vi "PH_PowerUnit_BaseClass.PC_EnablingState.vi"(0 "i ref in":refnum<vi>, 2 "Tagvalue":i32, 5 "error in (no error)":errorcluster) -> (14 "i ref out":refnum<vi>, 19 "error out":errorcluster)   [LabVIEW 2014, in "PH_PowerUnit_BaseClass.lvlib"]
doc: "This VI writes the Information from the PA Enabling Tag to own attributes and sets the GUI object."
uses:
  PH_PowerUnit_BaseClass.lvlib
  PH_SystemInformation/PH_SystemInformationEnabling State.ctl
  PH_SystemInformation/PH_SystemInformation.lvlib
  PH_Common/PH_Common.lvlib
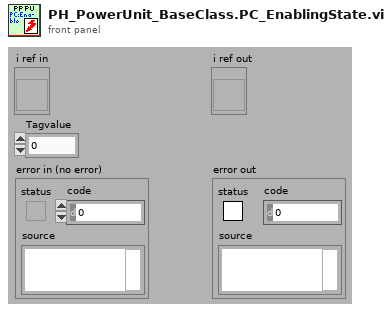
[diagram p1: front panel]
types:
  T1 = typedef "PH_PowerUnit_BaseClass.lvlib/PH_PowerUnit_BaseClass.i attribute.ctl" = cluster{"Constructor finished":bool, "PU":cluster{"In use":bool, "Service ID in use":i32, "GUI Ref":refnum<vi>}, "Enabling":cluster{"State":T2, "GUI Ref":refnum<vi>}, "Timing":cluster{"Last Shot":dbl, "Time between Shots [Sec]":dbl, "Waiting Time over?":bool, "Service ID Waiting Time":i32, "GUI Ref":refnum<vi>, "Instance":cluster{"Status":T3, "linked?":bool, "GUI Ref":refnum<vi>}}, "Sequencer":cluster{"SM State":string, "GUI Ref":refnum<vi>, "linked":bool}, "Subscribed Trendmssgs":cluster{"Tagname":string, "Status":T3, "linked?":bool, "Shot Condition":T3, "GUI Ref":refnum<vi>}[], "PP PU":T4, "Default Voltage (V)":dbl, "GUI Refs":T5, "PSDB data":cluster{"Shot Voltage [V]":dbl, "State TO SM":T6, "Write 2 early":bool}, "State TO SM":T6}
  T2 = typedef "PH_SystemInformation.lvlib/PH_SystemInformationEnabling State.ctl" = i32
  T3 = typedef "PH_StatusHandler.lvlib/PH_StatusHandler.Status.ctl" = i16
  T4 = typedef "PH_PP_Common.lvlib/PH_PP_Common.PUs.ctl" = enum16{"no Info", "PA-19mm-1", "PA-19mm-2", "PA-45mm-PILC", "PA-45mm-MAIN", "MA-PU-1", "MA-PU-2", "MA-PU-3", "MA-PU-4", "MA-PU-5", "MA-PU-6", "MA-FR", "MA-PILC", "PA-45mm-DP"}
  T5 = typedef "PH_PowerUnit_BaseClass.lvlib/PH_PowerUnit_BaseClass.GUI Refs.ctl" = cluster{"Delete Inst":refnum<vi>, "State TO SM":refnum<vi>, "State SM":refnum<vi>, "Fire":refnum<vi>}
  T6 = typedef "PH_PowerUnit_BaseClass.lvlib/PH_PowerUnit_BaseClass.SM States.ctl" = enum16{".", "Stand by", "Switch PU on", "Configure", "Set Default Voltage", "Set STANDBY", "Set READY", "Wait for Shot Cmd", "Open Dump Rods", "Open Ross Relais", "Close Ross Relais", "Switch PSU on", "Switch PSU off", "Charge", "Switch GD Channel on", "Close Dump Rods", "Rods-TO", "RR-TO", "PSU-TO", "Trigger-TO"}
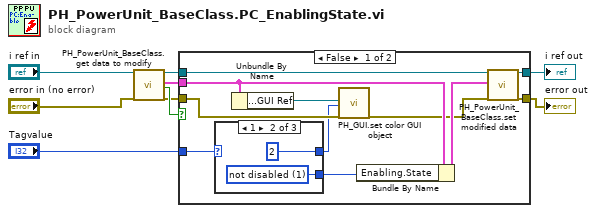
[diagram p0: block diagram]
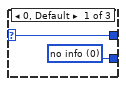
[diagram p2: hidden frame]
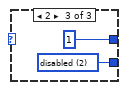
[diagram p3: hidden frame]
diagram:
  n1 = call "PH_PowerUnit_BaseClass.get data to modify.vi"("i ref in"="i ref in", "error in (no error)"="error in (no error)") -> ("i ref out"=w3:refnum<vi>, "i attribute"=w2:T1, "timed out"=w9:bool, "error out"=w5:errorcluster)  [unwired: 14 in]
  n2 = case shown="False" w9 {
    tunnel: w3 -> [w20 w28]
    tunnel: [w15 w28] -> w4
    tunnel: w5 -> [w12 w27]
    tunnel: [w14 w27] -> w6
    tunnel: w2 -> [w18 _]
    tunnel: "Tagvalue" -> [w17 _]
    frame False {
      n3 = case shown="1" w17 {
        selector: w17 -> [w22 _ _]
        tunnel: [w22 2 1 ("Numeric")] -> w10
        tunnel: [w21 w23 w25] -> w16
        frame 0, Default {
          w21 = T2 0 items=["no info", "not disabled", "disabled"] ("MainAmp Enabling State")
        }
        frame 1 {
          w23 = T2 1 items=["no info", "not disabled", "disabled"] ("MainAmp Enabling State")
        }
        frame 2 {
          w25 = T2 2 items=["no info", "not disabled", "disabled"] ("MainAmp Enabling State")
        }
      }
      n4 = Unbundle By Name(w18) -> ("Enabling.GUI Ref"=w13:refnum<vi>)
      n5 = call "PH_GUI.set color GUI object.vi"("GUI object Ref"=w13, "State"=w10, "error in (no error)"=w12) -> ("error out"=w11:errorcluster)  [unwired: 16 in]
      n6 = Bundle By Name(cluster=w18, "Enabling.State"=w16) -> (w19:T1)
      n7 = call "PH_PowerUnit_BaseClass.set modified data.vi"("i ref in"=w20, "i attribute"=w19, "error in (no error)"=w11) -> ("i ref out"=w15:refnum<vi>, "error out"=w14:errorcluster)  [unwired: 15 in]
    }
    frame True {
    }
  }
  "error out" <- w6
  "i ref out" <- w4
